vi "Oxford visa write read byte sized-- Hg.vi"(6 "milliseconds -- wait time":u32=11, 7 "byte count":u32=16, 8 "error in (no error)":errorcluster, 10 "write buffer":string, 11 "VISA resource name":refnum<visa-resource-name>) -> (0 "error out":errorcluster, 2 "read buffer":string, 3 "VISA resource name out":refnum<visa-resource-name>)   [LabVIEW 2015]
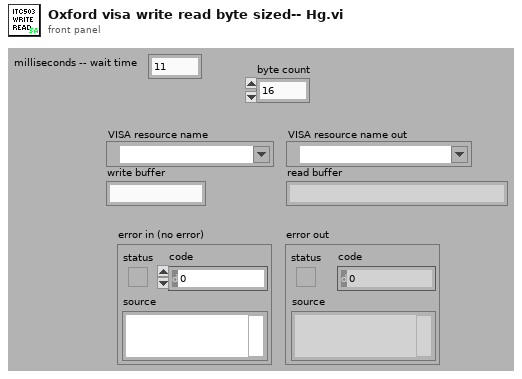
[diagram p1: front panel]
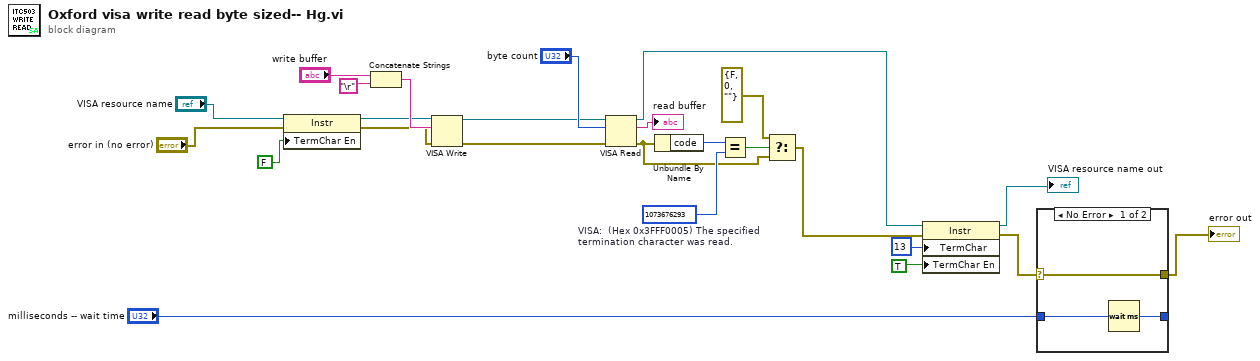
[diagram p0: block diagram]
diagram:
  w19 = 1073676293  # VISA:  (Hex 0x3FFF0005) The specified termination character was read.
  n1 = property class="Instr"(reference="VISA resource name", error in="error in (no error)", "TermChar En"=FALSE ("Message Based Settings:Termination Character Enable")) -> (reference out=w9:refnum<visa-resource-name>, error out=w10:errorcluster)
  n2 = Concatenate Strings("write buffer", "\r") -> (w22:string)
  n3 = VISA Write(VISA resource name=w9, write buffer=w22, error in (no error)=w10) -> (VISA resource name out=w15:refnum<visa-resource-name>, error out=w14:errorcluster)  [unwired: 1 out]
  n4 = VISA Read(VISA resource name=w15, byte count="byte count", error in (no error)=w14) -> (VISA resource name out=w5:refnum<visa-resource-name>, read buffer=→"read buffer":string, error out=w18:errorcluster)  [unwired: 1 out]
  n5 = Unbundle By Name(w18) -> ("code"=w20:i32)
  n6 = Equal?(x=w20, y=w19) -> (x = y?=w17:bool)
  n7 = Select(t=errorcluster {"status"=FALSE, "code"=0, "source"=""}, s=w17, f=w18) -> (s? t:f=w6:errorcluster)
  n8 = property class="Instr"(reference=w5, error in=w6, "TermChar"=u8 13 ("Message Based Settings:Termination Character"), "TermChar En"=TRUE ("Message Based Settings:Termination Character Enable")) -> (reference out=→"VISA resource name out":refnum<visa-resource-name>, error out=w3:errorcluster)
  n9 = case shown="No Error" w3 {
    selector: w3 -> [w28 w30]
    tunnel: [w28 w30] -> w2
    tunnel: "milliseconds -- wait time" -> [w27 w29]
    tunnel: [w26 w29] -> _
    frame No Error {
      n10 = Wait (ms)(milliseconds to wait=w27) -> (millisecond timer value=w26:u32)
    }
    frame Error {
    }
  }
  "error out" <- w2
